vi "Run Motion Profile V2.0.vi"   [LabVIEW 2017]
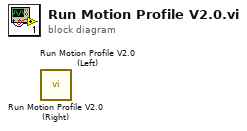
[diagram p0: block diagram]
diagram:
  n1 = call "Run Motion Profile V2.0 (Right).vi"() -> ()  [unwired: 12 in]
  n2 = call "Run Motion Profile V2.0 (Left).vi"() -> ()  [unwired: 12 in]
